vi "Array to Multi Ch Spectrums.vi"(8 "channel names":string[](array[string]), 9 "f0":dbl, 10 "df":dbl, 11 "array":dbl[](array[numeric])) -> (3 "spectra":cluster{"x0":dbl, "dx":dbl, "magnitude":dbl[]}[](array[cluster]))   [LabVIEW 2021]
uses:
  84c6873b-ba5f-40aa-b115-c7938ee3858f.vi
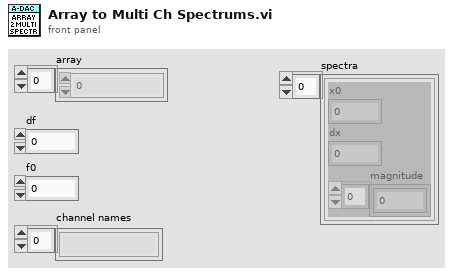
[diagram p1: front panel]
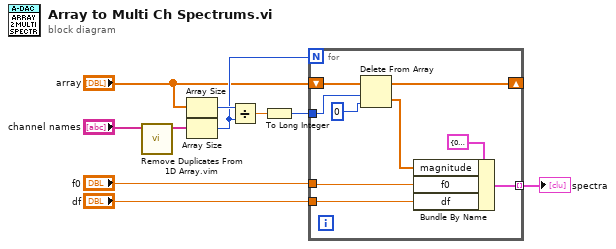
[diagram p0: block diagram]
diagram:
  n1 = call "Remove Duplicates From 1D Array.vim"("array"="channel names") -> ("array with duplicates removed"=w1:string[])  [unwired: 10 in]
  n2 = Array Size(array="array") -> (size(s)=w10:i32)
  n3 = Array Size(array=w1) -> (size(s)=w9:i32)
  n4 = Divide(x=w10, y=w9) -> (x/y=w7:dbl)
  n5 = To Long Integer(number=w7) -> (32bit integer=w6:i32)
  n6 = for {
    N: w9 -> [_]
    shift-right: [w18] -> _
    shift-left: "array" -> [w19]
    tunnel: w6 -> [w16]
    tunnel: "df" -> [w12]
    tunnel: [w15] -> w3 mode=indexing
    tunnel: "f0" -> [w13]
    n7 = Delete From Array(array=w19, length=w16, index=0) -> (deleted portion=w11:dbl[], array with subset deleted=w18:dbl[])
    n8 = Bundle By Name(cluster=cluster{"f0":dbl, "df":dbl, "magnitude":dbl[]} {"f0"=0.0, "df"=0.0, "magnitude"=[]} ("converted spectrum"), "magnitude"=w11, "f0"=w13, "df"=w12) -> (w15:cluster{"f0":dbl, "df":dbl, "magnitude":dbl[]})
  }
  "spectra" <- w3
